vi "mas ejemplos de for.vi"() -> ()   [LabVIEW 2020]
panel:
  out "Numeric":dbl
  out "Boolean":bool
  in  "String":string
  # "Escribir un programa que encuenda un leda cuando encuentre una letra \"a\" o \"A\"\n\n\n\n\n\nEscribir un programa que sume los números divisibles entre 2 y 5 del 100 al 200"
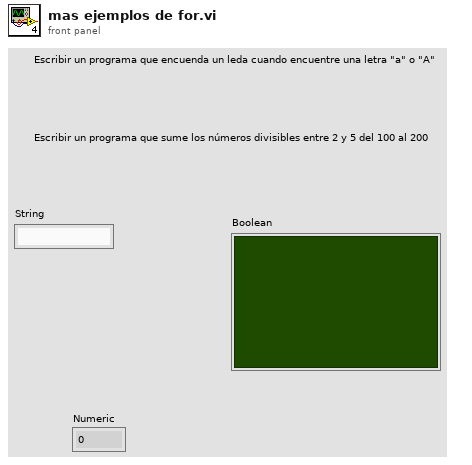
[diagram p1: front panel]
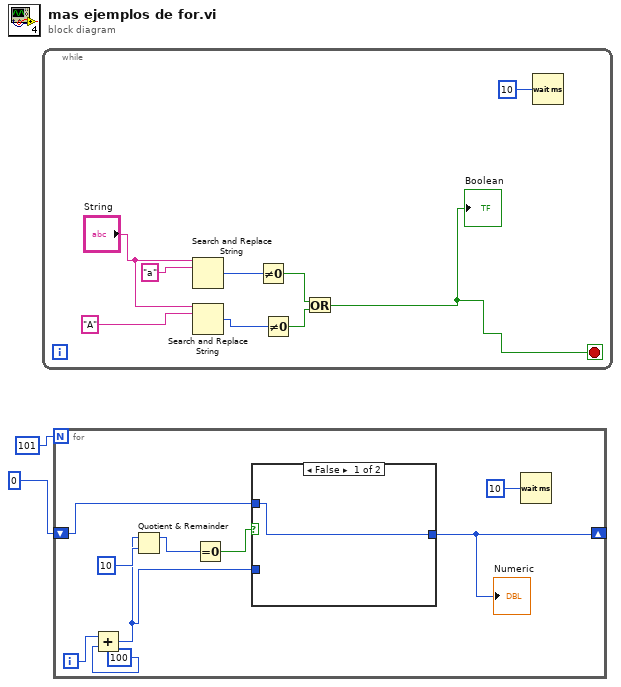
[diagram p0: block diagram]
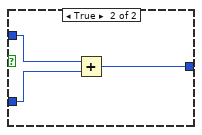
[diagram p2: hidden frame]
diagram:
  n1 = while {
    stop <- w5 stop-if-true
    n2 = Search and Replace String(input string="String", search string="a") -> (number of replacements=w8:i32)  [unwired: 6 in, 3 out]
    n3 = Search and Replace String(input string="String", search string="A") -> (number of replacements=w3:i32)  [unwired: 6 in, 3 out]
    n4 = Not Equal To 0?(x=w8) -> (x != 0?=w7:bool)
    n5 = Not Equal To 0?(x=w3) -> (x != 0?=w6:bool)
    n6 = Or(x=w7, y=w6) -> (x .or. y?=w5:bool)
    "Boolean" <- w5
    n7 = Wait (ms)(milliseconds to wait=10) -> ()  [unwired: 1 out]
  }
  n8 = for {
    N: 101 -> [_]
    shift-right: [w14] -> _
    shift-left: 0 -> [w12]
    i -> [w20]
    n9 = Add(x=w20, y=100) -> (x+y=w15:i32)
    n10 = Quotient & Remainder(x=w15, y=10) -> (x-y*floor(x/y)=w17:i32)  [unwired: 1 out]
    n11 = Equal To 0?(x=w17) -> (x = 0?=w16:bool)
    n12 = case shown="False" w16 {
      tunnel: w15 -> [_ w24]
      tunnel: [w21 w23] -> w14
      tunnel: w12 -> [w21 w22]
      frame False {
      }
      frame True {
        n13 = Add(x=w22, y=w24) -> (x+y=w23:i32)
      }
    }
    "Numeric" <- w14
    n14 = Wait (ms)(milliseconds to wait=10) -> ()  [unwired: 1 out]
  }
